vi "Express.vi"() -> (0 "Accelerometer":cluster{"Z":i16, "Y":i16, "X":i16} {"X" scale=-10.0..300.0; "Y" scale=-10.0..300.0; "Z" scale=-10.0..300.0})   [LabVIEW 2015]
uses:
  <vilib>/rvi/Emulation/niFpgaGetClockAttributes.vi
  <vilib>/rvi/Emulation/niFpgaSctlEmulationGetInTimedLoop.vi
  <vilib>/rvi/Emulation/niFpgaEmulationReportErrorSimple.vi
  <vilib>/rvi/eio/common/nirviEmuTemplateMethod_errors.vi
  <vilib>/rvi/Emulation/niFpgaCriticalErrorInLSC.vi
  <vilib>/eio/EIONode/EIONode.xnode
panel:
  in  "Arm":enum16{"meArm", "uArm"}(ring)
  in  "S3":u32(slide)=500 min=500 max=2500 scale=500.0..2500.0
  in  "S4":u32(slide)=500 min=500 max=2500 scale=500.0..2500.0
  in  "S2":u32(slide)=500 min=500 max=2500 scale=500.0..2500.0
  in  "S1":u32(slide)=500 min=500 max=2500 scale=500.0..2500.0
  in  "Frequency (Hz)":u32=5000
  in  "Motor Speed Right":i16(slide) scale=0.0..5.0
  in  "Motor Speed Left":i16(slide) scale=0.0..5.0
  in  "LED 3":T1 {"Brightness" max=1000}
  in  "LED 2":T2 {"Brightness" max=1000}
  in  "LED 1":T3 {"Brightness" max=1000}
  in  "LED 0":T4 {"Brightness" max=1000}
  in  "C5H":T5
  out "IR":cluster{"1":bool, "2":bool}
  in  "Mot F":T6
  out "Ultrasuond":cluster{"US BK":u32, "US FR":u32, "US FL":u32}
  out "Button":bool
  out "PIR":bool
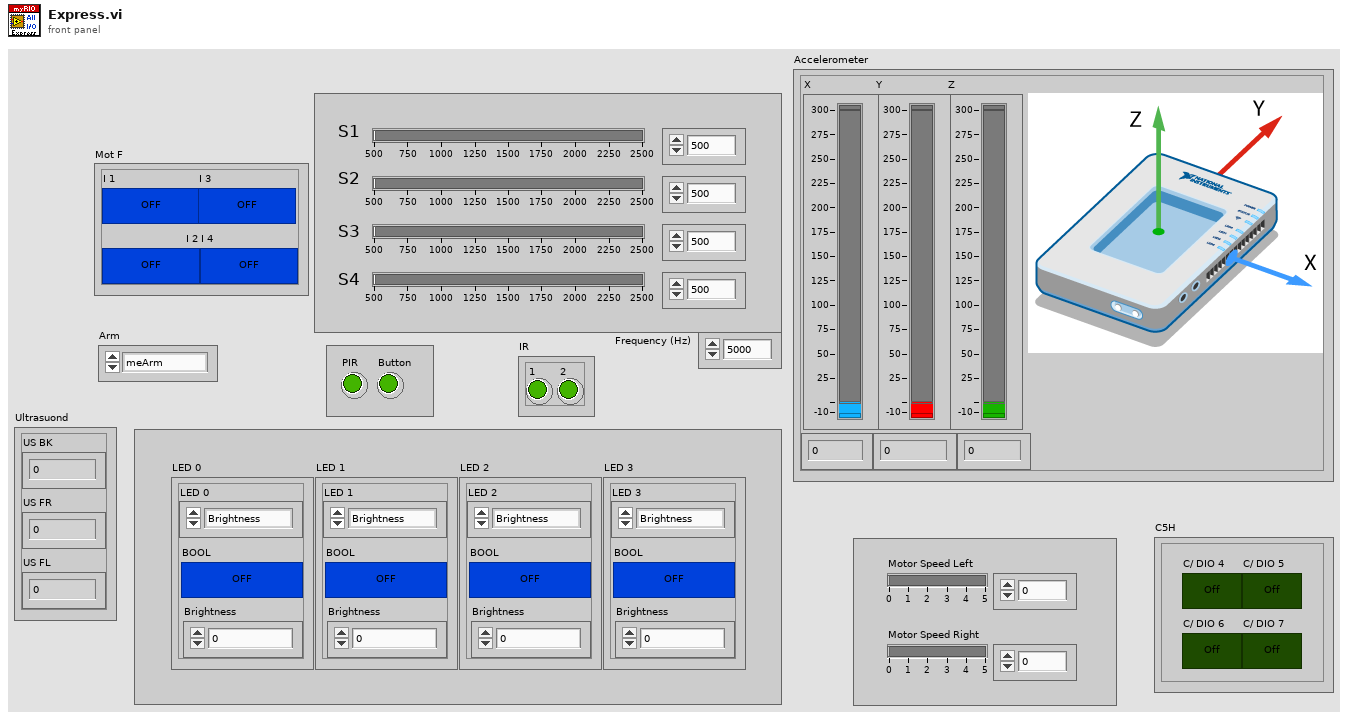
[diagram p1: front panel]
types:
  T1 = cluster{"LED 3":enum16{"Brightness", "Bool"}, "BOOL":bool, "Brightness":u32}
  T2 = cluster{"LED 2":enum16{"Brightness", "Bool"}, "BOOL":bool, "Brightness":u32}
  T3 = cluster{"LED 1":enum16{"Brightness", "Bool"}, "BOOL":bool, "Brightness":u32}
  T4 = cluster{"LED 0":enum16{"Brightness", "Bool"}, "BOOL":bool, "Brightness":u32}
  T5 = cluster{"C/ DIO 4":bool, "C/ DIO 5":bool, "C/ DIO 6":bool, "C/ DIO 7":bool}
  T6 = cluster{"I 1":bool, "I 2":bool, "I 3":bool, "I 4":bool}
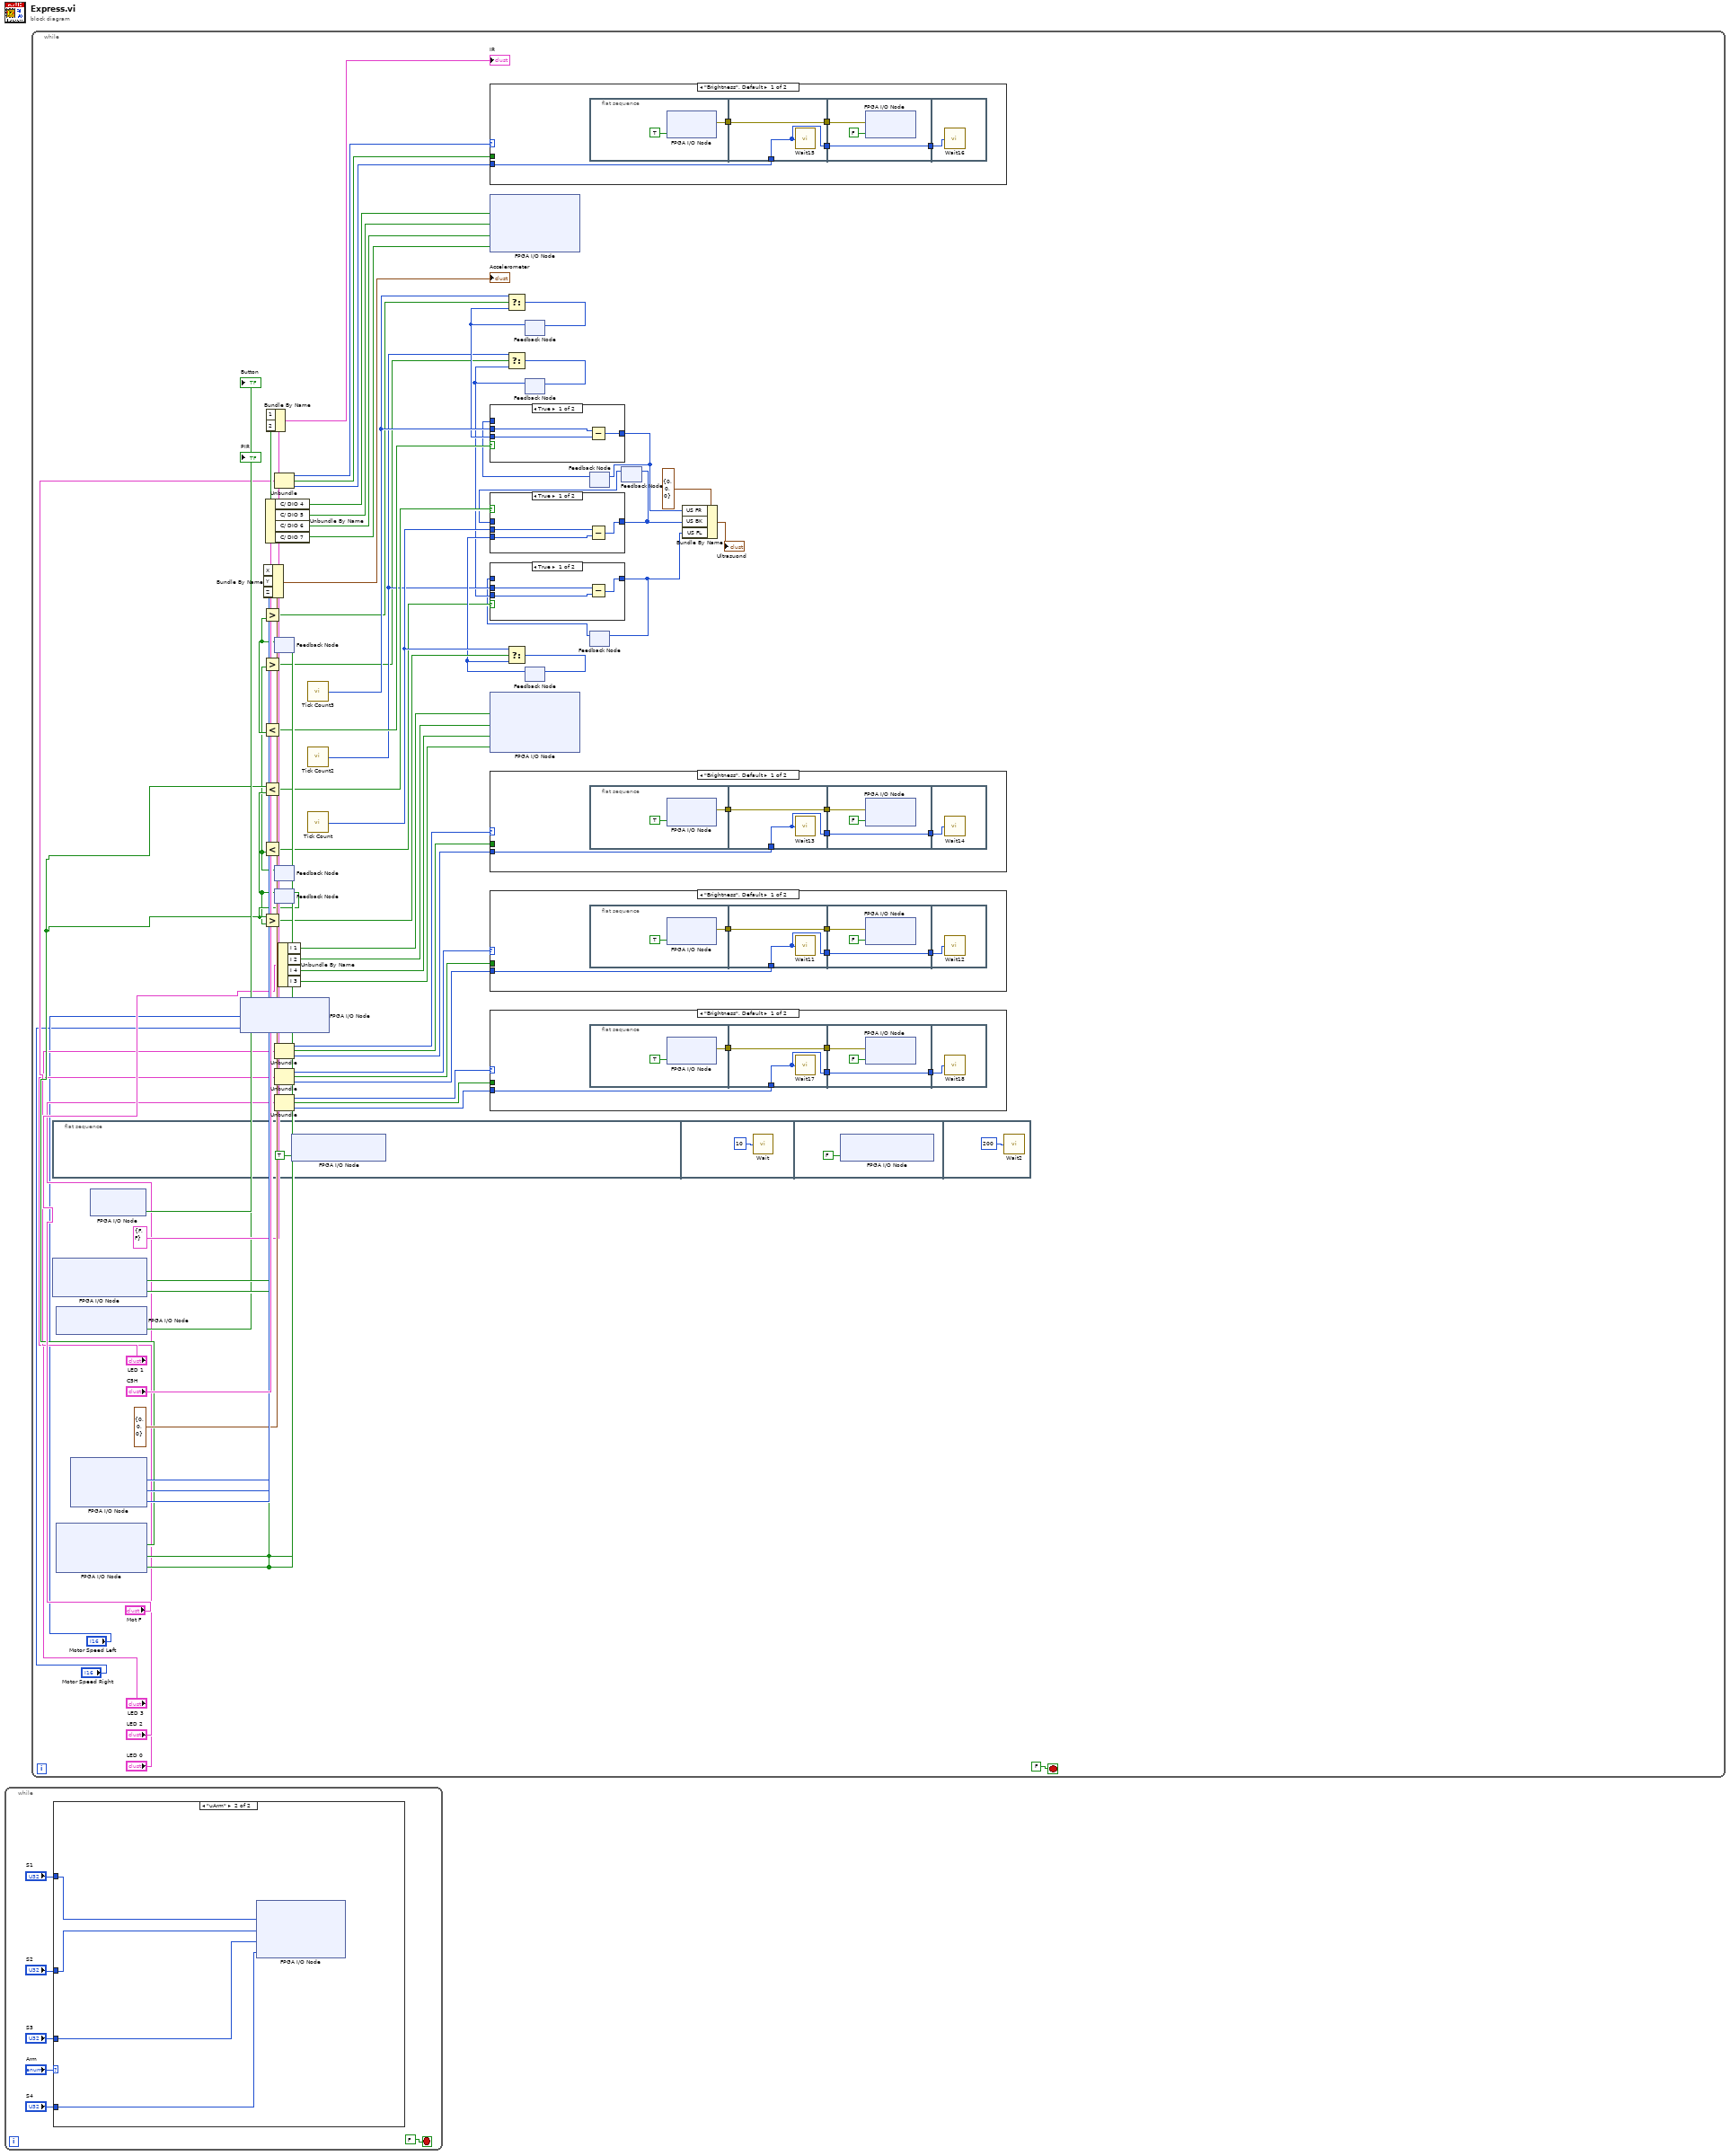
[diagram p0: block diagram]
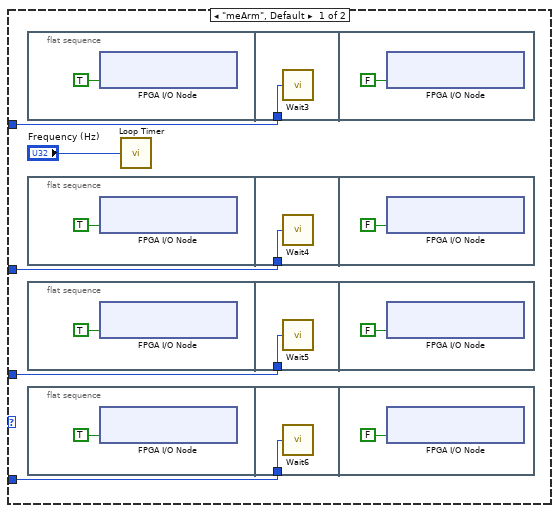
[diagram p2: hidden frame]
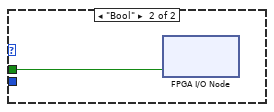
[diagram p3: hidden frame]
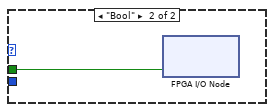
[diagram p4: hidden frame]
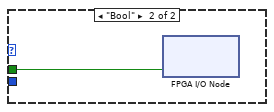
[diagram p5: hidden frame]
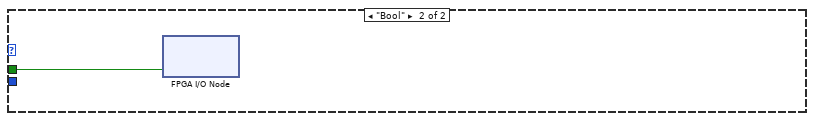
[diagram p6: hidden frame]
diagram:
  n1 = while {
    stop <- FALSE stop-if-true
    n2 = case shown="\"uArm\"" "Arm" {
      tunnel: "S1" -> [w10 w27]
      tunnel: "S2" -> [w9 w26]
      tunnel: "S3" -> [w8 w25]
      tunnel: "S4" -> [w7 w24]
      frame "meArm", Default {
        n3 = flat-sequence {
          tunnel: w10 -> [w13]
          frame #0 {
            n4 = xnode "FPGA I/O Node"("ConnectorB/DIO0"=TRUE) -> ()  [unwired: 1 in, 1 out]
          }
          frame #1 {
            n5 = call "Wait3"("Count(uSec)"=w13) -> ()  [unwired: 1 out]
          }
          frame #2 {
            n6 = xnode "FPGA I/O Node"("ConnectorB/DIO0"=FALSE) -> ()  [unwired: 1 in, 1 out]
          }
        }
        n7 = flat-sequence {
          tunnel: w9 -> [w16]
          frame #0 {
            n8 = xnode "FPGA I/O Node"("ConnectorB/DIO1"=TRUE) -> ()  [unwired: 1 in, 1 out]
          }
          frame #1 {
            n9 = call "Wait4"("Count(uSec)"=w16) -> ()  [unwired: 1 out]
          }
          frame #2 {
            n10 = xnode "FPGA I/O Node"("ConnectorB/DIO1"=FALSE) -> ()  [unwired: 1 in, 1 out]
          }
        }
        n11 = flat-sequence {
          tunnel: w8 -> [w19]
          frame #0 {
            n12 = xnode "FPGA I/O Node"("ConnectorB/DIO2"=TRUE) -> ()  [unwired: 1 in, 1 out]
          }
          frame #1 {
            n13 = call "Wait5"("Count(uSec)"=w19) -> ()  [unwired: 1 out]
          }
          frame #2 {
            n14 = xnode "FPGA I/O Node"("ConnectorB/DIO2"=FALSE) -> ()  [unwired: 1 in, 1 out]
          }
        }
        n15 = flat-sequence {
          tunnel: w7 -> [w22]
          frame #0 {
            n16 = xnode "FPGA I/O Node"("ConnectorB/DIO3"=TRUE) -> ()  [unwired: 1 in, 1 out]
          }
          frame #1 {
            n17 = call "Wait6"("Count(uSec)"=w22) -> ()  [unwired: 1 out]
          }
          frame #2 {
            n18 = xnode "FPGA I/O Node"("ConnectorB/DIO3"=FALSE) -> ()  [unwired: 1 in, 1 out]
          }
        }
        n19 = call "Loop Timer"("Count(uSec)"="Frequency (Hz)") -> ()  [unwired: 1 out]
      }
      frame "uArm" {
        n20 = xnode "FPGA I/O Node"("ConnectorA/AO0"=w27, "ConnectorA/AO1"=w26, "ConnectorB/AO0"=w25, "ConnectorB/AO1"=w24) -> ()  [unwired: 4 in, 4 out]
      }
    }
  }
  n21 = while {
    stop <- FALSE stop-if-true
    n22 = flat-sequence {
      frame #0 {
        n23 = xnode "FPGA I/O Node"("ConnectorA/DIO11"=TRUE ("ConnectorC/DIO6")) -> ()  [unwired: 2 in, 2 out]
      }
      frame #1 {
        n24 = call "Wait"("Count(uSec)"=u32 10) -> ()  [unwired: 1 out]
      }
      frame #2 {
        n25 = xnode "FPGA I/O Node"("ConnectorA/DIO11"=FALSE ("ConnectorC/DIO6")) -> ()  [unwired: 2 in, 2 out]
      }
      frame #3 {
        n26 = call "Wait2"("Count(uSec)"=u32 200 ("Trigger pulse interval (mSec)")) -> ()  [unwired: 1 out]
      }
    }
    n27 = xnode "FPGA I/O Node"() -> ("ConnectorA/DIO13"=w81:bool, "ConnectorA/DIO14"=w82:bool)  [unwired: 3 in, 3 out]
    n28 = xnode "FPGA I/O Node"() -> ("ConnectorA/DIO4"=→"PIR":bool)  [unwired: 2 in, 2 out]
    n29 = xnode "FPGA I/O Node"() -> ("ConnectorA/DIO5"=w62:bool, "ConnectorA/DIO6"=w71:bool, "ConnectorA/DIO7"=w72:bool)  [unwired: 4 in, 4 out]
    n30 = xnode "FPGA I/O Node"() -> ("AccelerationX"=w85:i16, "AccelerationY"=w86:i16, "AccelerationZ"=w87:i16)  [unwired: 4 in, 4 out]
    n31 = xnode "FPGA I/O Node"() -> ("Button0"=→"Button":bool)  [unwired: 2 in, 2 out]
    n32 = xnode "FPGA I/O Node"("ConnectorC/AO0"="Motor Speed Left", "ConnectorC/AO1"="Motor Speed Right") -> ()  [unwired: 2 in, 2 out]
    n33 = Bundle By Name(cluster=cluster{"Z":i16, "Y":i16, "X":i16} {"Z"=0, "Y"=0, "X"=0} ("Accelerometer"), "X"=w85, "Y"=w86, "Z"=w87) -> (→"Accelerometer":cluster{"Z":i16, "Y":i16, "X":i16})
    n34 = Unbundle By Name("C5H") -> ("C/ DIO 4"=w93:bool, "C/ DIO 5"=w94:bool, "C/ DIO 6"=w95:bool, "C/ DIO 7"=w96:bool)
    n35 = Bundle By Name(cluster=cluster{"1":bool, "2":bool} {"1"=FALSE, "2"=FALSE} ("IR"), "1"=w81, "2"=w82) -> (→"IR":cluster{"1":bool, "2":bool})
    n36 = Unbundle("LED 1") -> ("LED 1"=w44:enum16{"Brightness", "Bool"}, "BOOL"=w42:bool, "Brightness"=w43:u32)
    n37 = feedback #1() -> (w68:bool)  [unwired: 1 in]
    n38 = Greater?(x=w71, y=w68) -> (0:w67:bool)
    n39 = Less?(x=w71, y=w68) -> (x < y?=w69:bool)
    n40 = feedback-in #1(w71) -> ()
    n41 = feedback #2() -> (w53:bool)  [unwired: 1 in]
    n42 = Greater?(x=w72, y=w53) -> (0:w52:bool)
    n43 = Less?(x=w72, y=w53) -> (x < y?=w54:bool)
    n44 = feedback-in #2(w72) -> ()
    n45 = feedback #3() -> (w60:bool)  [unwired: 1 in]
    n46 = Less?(x=w62, y=w60) -> (x < y?=w61:bool)
    n47 = Greater?(x=w62, y=w60) -> (0:w59:bool)
    n48 = feedback-in #3(w62) -> ()
    n49 = Unbundle("LED 3") -> ("LED 3"=w33:enum16{"Brightness", "Bool"}, "BOOL"=w41:bool, "Brightness"=w36:u32)
    n50 = Unbundle("LED 2") -> ("LED 2"=w34:enum16{"Brightness", "Bool"}, "BOOL"=w40:bool, "Brightness"=w37:u32)
    n51 = Unbundle("LED 0") -> ("LED 0"=w35:enum16{"Brightness", "Bool"}, "BOOL"=w39:bool, "Brightness"=w38:u32)
    n52 = Unbundle By Name("Mot F") -> ("I 1"=w73:bool, "I 2"=w74:bool, "I 4"=w75:bool, "I 3"=w76:bool)
    n53 = call "Tick Count3"() -> ("Tick Count(uSec)"=w70:u32)
    n54 = call "Tick Count2"() -> ("Tick Count(uSec)"=w55:u32)
    n55 = call "Tick Count"() -> ("Tick Count(uSec)"=w63:u32)
    n56 = case shown="\"Brightness\", Default" w44 {
      tunnel: w43 -> [w141 _]
      tunnel: w42 -> [_ w152]
      frame "Brightness", Default {
        n57 = flat-sequence {
          tunnel: [w144] -> w143
          tunnel: [w147] -> w142
          tunnel: w143 -> [w147]
          tunnel: w141 -> [w146]
          tunnel: [w146] -> w139
          tunnel: w142 -> [w149]
          tunnel: [w148] -> w140
          tunnel: w139 -> [w148]
          tunnel: w140 -> [w151]
          frame #0 {
            n58 = xnode "FPGA I/O Node"("LED1"=TRUE) -> ("error out"=w144:errorcluster)  [unwired: 2 in, 1 out]
          }
          frame #1 {
            n59 = call "Wait15"("Count(uSec)"=w146) -> ()  [unwired: 1 out]
          }
          frame #2 {
            n60 = xnode "FPGA I/O Node"("error in"=w149, "LED1"=FALSE) -> ()  [unwired: 1 in, 2 out]
          }
          frame #3 {
            n61 = call "Wait16"("Count(uSec)"=w151) -> ()  [unwired: 1 out]
          }
        }
      }
      frame "Bool" {
        n62 = xnode "FPGA I/O Node"("LED1"=w152) -> ()  [unwired: 2 in, 2 out]
      }
    }
    n63 = xnode "FPGA I/O Node"("ConnectorC/DIO4"=w93, "ConnectorC/DIO5"=w94, "ConnectorC/DIO6"=w95, "ConnectorC/DIO7"=w96) -> ()  [unwired: 4 in, 4 out]
    n64 = xnode "FPGA I/O Node"("ConnectorA/DIO0"=w73, "ConnectorA/DIO1"=w74, "ConnectorA/DIO2"=w75, "ConnectorA/DIO3"=w76) -> ()  [unwired: 5 in, 5 out]
    n65 = case shown="\"Brightness\", Default" w33 {
      tunnel: w36 -> [w127 _]
      tunnel: w41 -> [_ w138]
      frame "Brightness", Default {
        n66 = flat-sequence {
          tunnel: [w130] -> w129
          tunnel: [w133] -> w128
          tunnel: w129 -> [w133]
          tunnel: w127 -> [w132]
          tunnel: [w132] -> w125
          tunnel: w128 -> [w135]
          tunnel: [w134] -> w126
          tunnel: w125 -> [w134]
          tunnel: w126 -> [w137]
          frame #0 {
            n67 = xnode "FPGA I/O Node"("LED3"=TRUE) -> ("error out"=w130:errorcluster)  [unwired: 2 in, 1 out]
          }
          frame #1 {
            n68 = call "Wait13"("Count(uSec)"=w132) -> ()  [unwired: 1 out]
          }
          frame #2 {
            n69 = xnode "FPGA I/O Node"("error in"=w135, "LED3"=FALSE) -> ()  [unwired: 1 in, 2 out]
          }
          frame #3 {
            n70 = call "Wait14"("Count(uSec)"=w137) -> ()  [unwired: 1 out]
          }
        }
      }
      frame "Bool" {
        n71 = xnode "FPGA I/O Node"("LED3"=w138) -> ()  [unwired: 2 in, 2 out]
      }
    }
    n72 = case shown="\"Brightness\", Default" w34 {
      tunnel: w37 -> [w113 _]
      tunnel: w40 -> [_ w124]
      frame "Brightness", Default {
        n73 = flat-sequence {
          tunnel: [w116] -> w115
          tunnel: [w119] -> w114
          tunnel: w115 -> [w119]
          tunnel: w113 -> [w118]
          tunnel: [w118] -> w111
          tunnel: w114 -> [w121]
          tunnel: [w120] -> w112
          tunnel: w111 -> [w120]
          tunnel: w112 -> [w123]
          frame #0 {
            n74 = xnode "FPGA I/O Node"("LED2"=TRUE) -> ("error out"=w116:errorcluster)  [unwired: 2 in, 1 out]
          }
          frame #1 {
            n75 = call "Wait11"("Count(uSec)"=w118) -> ()  [unwired: 1 out]
          }
          frame #2 {
            n76 = xnode "FPGA I/O Node"("error in"=w121, "LED2"=FALSE) -> ()  [unwired: 1 in, 2 out]
          }
          frame #3 {
            n77 = call "Wait12"("Count(uSec)"=w123) -> ()  [unwired: 1 out]
          }
        }
      }
      frame "Bool" {
        n78 = xnode "FPGA I/O Node"("LED2"=w124) -> ()  [unwired: 2 in, 2 out]
      }
    }
    n79 = case shown="\"Brightness\", Default" w35 {
      tunnel: w38 -> [w99 _]
      tunnel: w39 -> [_ w110]
      frame "Brightness", Default {
        n80 = flat-sequence {
          tunnel: [w102] -> w101
          tunnel: [w105] -> w100
          tunnel: w101 -> [w105]
          tunnel: w99 -> [w104]
          tunnel: [w104] -> w97
          tunnel: w100 -> [w107]
          tunnel: [w106] -> w98
          tunnel: w97 -> [w106]
          tunnel: w98 -> [w109]
          frame #0 {
            n81 = xnode "FPGA I/O Node"("LED0"=TRUE) -> ("error out"=w102:errorcluster)  [unwired: 2 in, 1 out]
          }
          frame #1 {
            n82 = call "Wait17"("Count(uSec)"=w104) -> ()  [unwired: 1 out]
          }
          frame #2 {
            n83 = xnode "FPGA I/O Node"("error in"=w107, "LED0"=FALSE) -> ()  [unwired: 1 in, 2 out]
          }
          frame #3 {
            n84 = call "Wait18"("Count(uSec)"=w109) -> ()  [unwired: 1 out]
          }
        }
      }
      frame "Bool" {
        n85 = xnode "FPGA I/O Node"("LED0"=w110) -> ()  [unwired: 2 in, 2 out]
      }
    }
    n86 = feedback #4() -> (w65:u32)  [unwired: 1 in]
    n87 = Select(t=w70, s=w67, f=w65) -> (s? t:f=w66:u32)
    n88 = feedback-in #4(w66) -> ()
    n89 = feedback #5() -> (w50:u32)  [unwired: 1 in]
    n90 = Select(t=w55, s=w52, f=w50) -> (s? t:f=w51:u32)
    n91 = feedback-in #5(w51) -> ()
    n92 = feedback #6() -> (w57:u32)  [unwired: 1 in]
    n93 = Select(t=w63, s=w59, f=w57) -> (s? t:f=w58:u32)
    n94 = feedback-in #6(w58) -> ()
    n95 = feedback #7() -> (w64:u32)  [unwired: 1 in]
    n96 = case shown="True" w69 {
      tunnel: w64 -> [_ w156]
      tunnel: w70 -> [w153 _]
      tunnel: w65 -> [w154 _]
      tunnel: [w155 w156] -> w91
      frame True {
        n97 = Subtract(x=w153, y=w154) -> (x-y=w155:u32)
      }
      frame False {
      }
    }
    n98 = feedback-in #7(w91) -> ()
    n99 = feedback #8() -> (w49:u32)  [unwired: 1 in]
    n100 = case shown="True" w54 {
      tunnel: w49 -> [_ w164]
      tunnel: w55 -> [w161 _]
      tunnel: w50 -> [w162 _]
      tunnel: [w163 w164] -> w89
      frame True {
        n101 = Subtract(x=w161, y=w162) -> (x-y=w163:u32)
      }
      frame False {
      }
    }
    n102 = feedback-in #8(w89) -> ()
    n103 = feedback #9() -> (w56:u32)  [unwired: 1 in]
    n104 = case shown="True" w61 {
      tunnel: w56 -> [_ w160]
      tunnel: w63 -> [w157 _]
      tunnel: w57 -> [w158 _]
      tunnel: [w159 w160] -> w90
      frame True {
        n105 = Subtract(x=w157, y=w158) -> (x-y=w159:u32)
      }
      frame False {
      }
    }
    n106 = feedback-in #9(w90) -> ()
    n107 = Bundle By Name(cluster=cluster{"US BK":u32, "US FR":u32, "US FL":u32} {"US BK"=0, "US FR"=0, "US FL"=0} ("Ultrasuond"), "US FR"=w91, "US BK"=w90, "US FL"=w89) -> (→"Ultrasuond":cluster{"US BK":u32, "US FR":u32, "US FL":u32})
  }
